vi "ultraG.vi"() -> ()   [LabVIEW 2019]
panel:
  out "ultrasonic":dbl
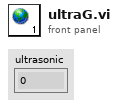
[diagram p1: front panel]
diagram:
